vi "NI_USB6343_DAQmx_AO_Test.vi"() -> ()   [LabVIEW 2020]
uses:
  <vilib>/DAQmx/write.llb/DAQmx Write (Analog 1D Wfm NChan NSamp).vi
  <vilib>/DAQmx/create/channels.llb/DAQmx Create Channel (AO-Voltage-Basic).vi
  <vilib>/DAQmx/configure/timing.llb/DAQmx Timing (Sample Clock).vi
  <vilib>/DAQmx/miscellaneous.llb/DAQmx Fill In Error Info.vi
  <resource>/objmgr/daqmx.rc
  <vilib>/measure/NI_MABase.lvlib
panel:
  out "Waveform Graph":waveform(dbl)(graph)
  out "error out":errorcluster
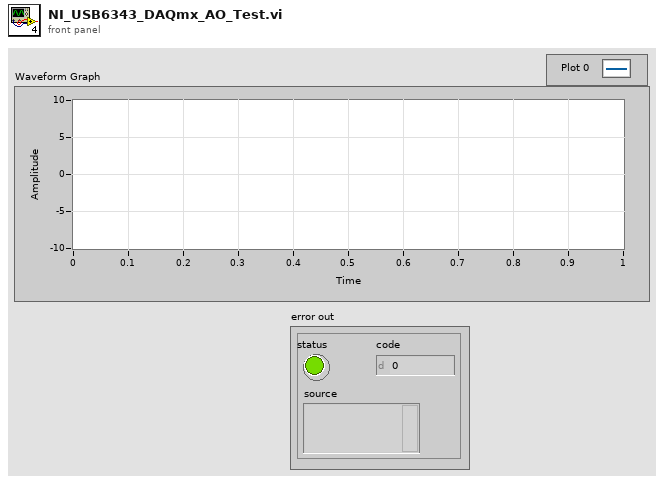
[diagram p1: front panel]
types:
  T1 = enum16{"Sine Wave", "Triangle Wave", "Square Wave", "Sawtooth Wave"}
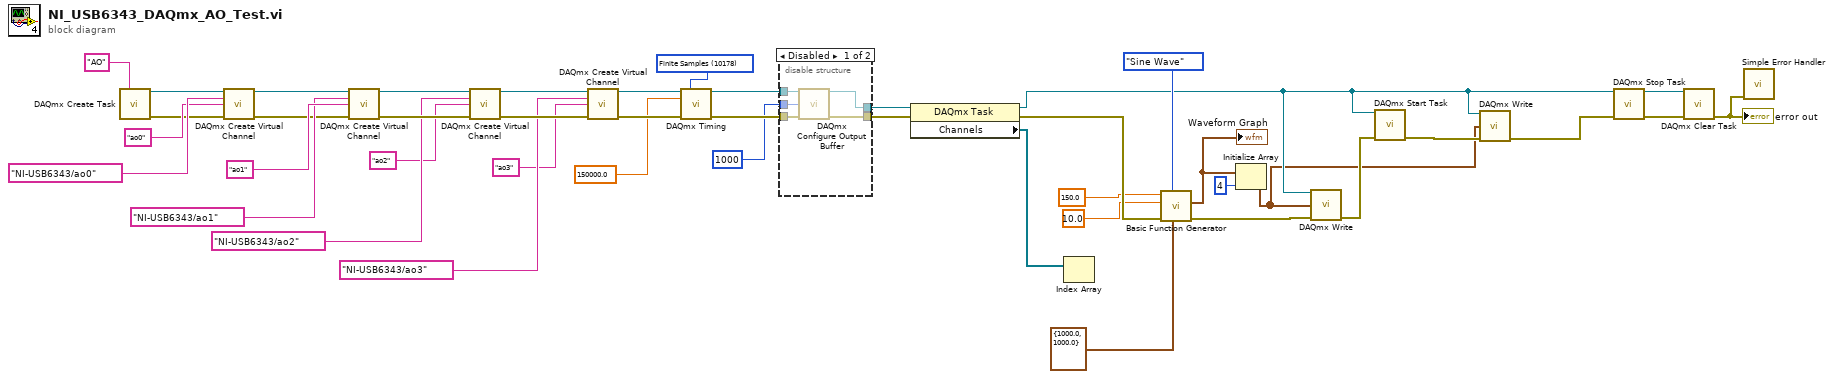
[diagram p0: block diagram]
diagram:
  w20 = 10178 items=["Finite Samples"=10178, "Continuous Samples"=10123, "Hardware Timed Single Point"=12522] ("sample mode")
  n1 = call <vilib>:"DAQmx Create Task.vi"("new task name"="AO") -> ("task out"=w42:refnum<k21>, "error out"=w36:errorcluster)  [unwired: 13 in]
  n2 = call-poly <vilib>:"DAQmx Create Virtual Channel.vi"("task in"=w42, "physical channels"=tag "NI-USB6343/ao0", "name to assign"="ao0", "error in"=w36) -> ("task out"=w39:refnum<k21>, "error out"=w35:errorcluster)  [unwired: 10 in]
  n3 = call-poly <vilib>:"DAQmx Create Virtual Channel.vi"("task in"=w39, "physical channels"=tag "NI-USB6343/ao1", "name to assign"="ao1", "error in"=w35) -> ("task out"=w33:refnum<k21>, "error out"=w34:errorcluster)  [unwired: 10 in]
  n4 = call-poly <vilib>:"DAQmx Create Virtual Channel.vi"("task in"=w33, "physical channels"=tag "NI-USB6343/ao2", "name to assign"="ao2", "error in"=w34) -> ("task out"=w28:refnum<k21>, "error out"=w27:errorcluster)  [unwired: 10 in]
  n5 = call-poly <vilib>:"DAQmx Create Virtual Channel.vi"("task in"=w28, "physical channels"=tag "NI-USB6343/ao3", "name to assign"="ao3", "error in"=w27) -> ("task out"=w22:refnum<k21>, "error out"=w21:errorcluster)  [unwired: 10 in]
  n6 = call-poly <vilib>:"DAQmx Timing.vi"("task/channels in"=w22, "sample mode"=w20, "rate"=150000.0, "error in"=w21) -> ("task out"=w12:refnum<k21>, "error out"=w11:errorcluster)  [unwired: 10 in]
  n7 = disable-structure shown="Disabled" {
    disable-tunnel: w12 -> [w48 w49]
    disable-tunnel: w11 -> [w47 w50]
    disable-tunnel: u32 1000 ("buffer size (in samples per channel)") -> [w46 _]
    disable-tunnel: [w45 w50] -> w9
    disable-tunnel: [w44 w49] -> w7
    frame Disabled {
      n8 = call <vilib>:"DAQmx Configure Output Buffer.vi"("task/channels in"=w48, "buffer size (in samples per channel)"=w46, "error in"=w47) -> ("task out"=w44:refnum<k21>, "error out"=w45:errorcluster)  [unwired: 11 in]
    }
    frame Enabled {
    }
  }
  n9 = property class="DAQmx Task"(reference=w7, error in=w9) -> (reference out=w4:refnum<k21>, error out=w18:errorcluster, "Channels"=w23:refnum<k21>[])
  n10 = Index Array(array=w23) -> ()  [unwired: 1 in, 1 out]
  n11 = call <vilib>:"Basic Function Generator.vi"("sampling info"=cluster{"Fs":dbl, "#s":dbl} {"Fs"=1000.0, "#s"=1000.0}, "signal type"=T1."Sine Wave", "error in (no error)"=w18, "amplitude"=10.0, "frequency"=150.0) -> ("error out"=w13:errorcluster, "signal out"=w5:waveform(dbl))  [unwired: 4 in, 1 out]
  "Waveform Graph" <- w5
  n12 = Initialize Array(w5, 4 ("dimension size")) -> (w1:waveform(dbl)[])
  n13 = call-poly <vilib>:"DAQmx Write.vi"("task/channels in"=w4, "data"=w1, "error in"=w13) -> ("error out"=w8:errorcluster)  [unwired: 10 in, 2 out]
  n14 = call <vilib>:"DAQmx Start Task.vi"("task/channels in"=w4, "error in"=w8) -> ("error out"=w3:errorcluster)  [unwired: 12 in, 1 out]
  n15 = call-poly <vilib>:"DAQmx Write.vi"("task/channels in"=w4, "data"=w1, "error in"=w3) -> ("error out"=w2:errorcluster)  [unwired: 10 in, 2 out]
  n16 = call <vilib>:"DAQmx Stop Task.vi"("task/channels in"=w4, "error in"=w2) -> ("task out"=w30:refnum<k21>, "error out"=w29:errorcluster)  [unwired: 12 in]
  n17 = call <vilib>:"DAQmx Clear Task.vi"("task in"=w30, "error in"=w29) -> ("error out"=w24:errorcluster)  [unwired: 13 in]
  "error out" <- w24
  n18 = call <vilib>:"Simple Error Handler.vi"("error in (no error)"=w24) -> ()  [unwired: 4 in, 5 out]
